vi "pb_inst_direct.vi"(8 "error in (no error)":errorcluster, 10 "PulseBlaster\nVLIW":T1, 11 "path in":path=path "C:/Program Files/SpinCore/SpinAPI/dll/spinapi.dll") -> (0 "error out":errorcluster, 3 "path out":path)   [LabVIEW 2013, in "SpinAPI-Interface.lvlib"]
uses:
  SpinAPI-Interface.lvlib
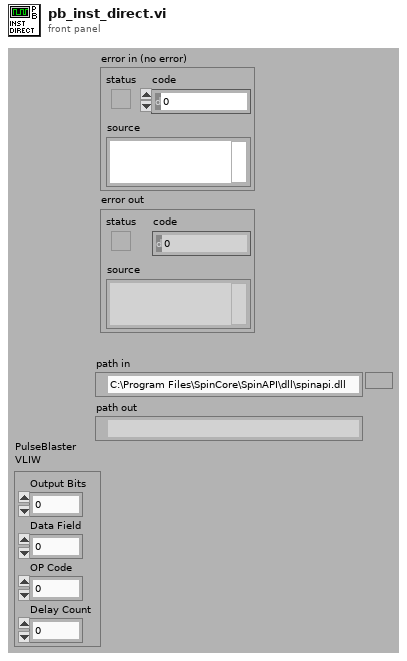
[diagram p1: front panel]
types:
  T1 = cluster{"Output Bits":u32, "Data Field":u32, "OP Code":u8, "Delay Count":u64}
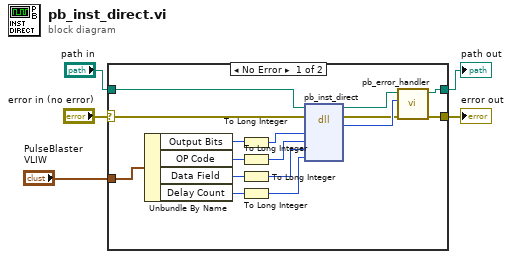
[diagram p0: block diagram]
diagram:
  n1 = case shown="No Error" "error in (no error)" {
    selector: "error in (no error)" -> [w20 w23]
    tunnel: [w15 w23] -> w5
    tunnel: "path in" -> [w19 w22]
    tunnel: [w16 w22] -> w2
    tunnel: "PulseBlaster\nVLIW" -> [w14 _]
    frame No Error {
      n2 = Unbundle By Name(w14) -> ("Output Bits"=w13:u32, "OP Code"=w10:u8, "Data Field"=w11:u32, "Delay Count"=w12:u64)
      n3 = To Long Integer(number=w13) -> (32bit integer=w9:i32)
      n4 = To Long Integer(number=w10) -> (32bit integer=w8:i32)
      n5 = To Long Integer(number=w11) -> (32bit integer=w7:i32)
      n6 = To Long Integer(number=w12) -> (32bit integer=w6:i32)
      n7 = dll-call lib="C:/SpinCore/SpinAPI/dll/spinapi.dll" fn="pb_inst_direct"(path in=w19, error in=w20, "flags"=w9, "inst"=w8, "inst_data"=w7, "length"=w6) -> (path out=w18:path, error out=w17:errorcluster, "return type"=w21:i32)  [unwired: 5 in]
      n8 = call "pb_error_handler.vi"("error in (no error)"=w17, "return code"=w21, "path in"=w18) -> ("error out"=w15:errorcluster, "path out"=w16:path)  [unwired: 7 out]
    }
    frame Error {
    }
  }
  "error out" <- w5
  "path out" <- w2
